vi "Query_Pelletron_Status.vi"(8 "error in (no error)":errorcluster, 10 "Read Selector":T1 items=["Facility Key", "Chain Bypass", "Rotating Shaft Bypass", "Facility Interlock", "Pressure Interlock", "Temperature Interlock", "Water Flow Interlock", "Blower Status", "High Voltage", "+ High Voltage PS Readout", "- High Voltage PS Readout", "High Voltage PS Setting", "Ion Gauge", "Ion Filament", "Control Reference Voltage", "Control Mode", "Power Supply", "Chain Current", "Column Current", "Lost Current", "High Voltage Power Supply", "Rotating Shaft", "Chain", "Beamline GV", "Radiation", "Spark Count", "Spark Limit", "Spark Interlock", "Spark Threshold", "HV Difference from Control"], 11 "AccelNET.lvlib:TCP.lvclass":refnum<class "TCP.lvclass">) -> (0 "error out":errorcluster, 2 "Data Out":dbl)   [LabVIEW 2012, in "AccelNET.lvlib" / "TCP.lvclass"]
uses:
  TCP.lvclass
  Read_Selector.ctl
  TCP.lvclass/TCP.ctl
  Useful_Controls.lvlib
panel:
  out "substring":string
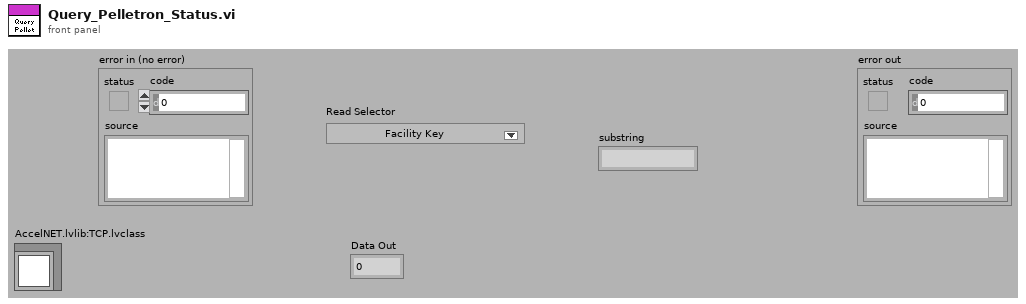
[diagram p1: front panel]
types:
  T1 = typedef "AccelNET.lvlib/Useful_Controls.lvlib/Read_Selector.ctl" = u16
  T2 = enum16{"Standard", "Buffered", "CRLF", "Immediate"}
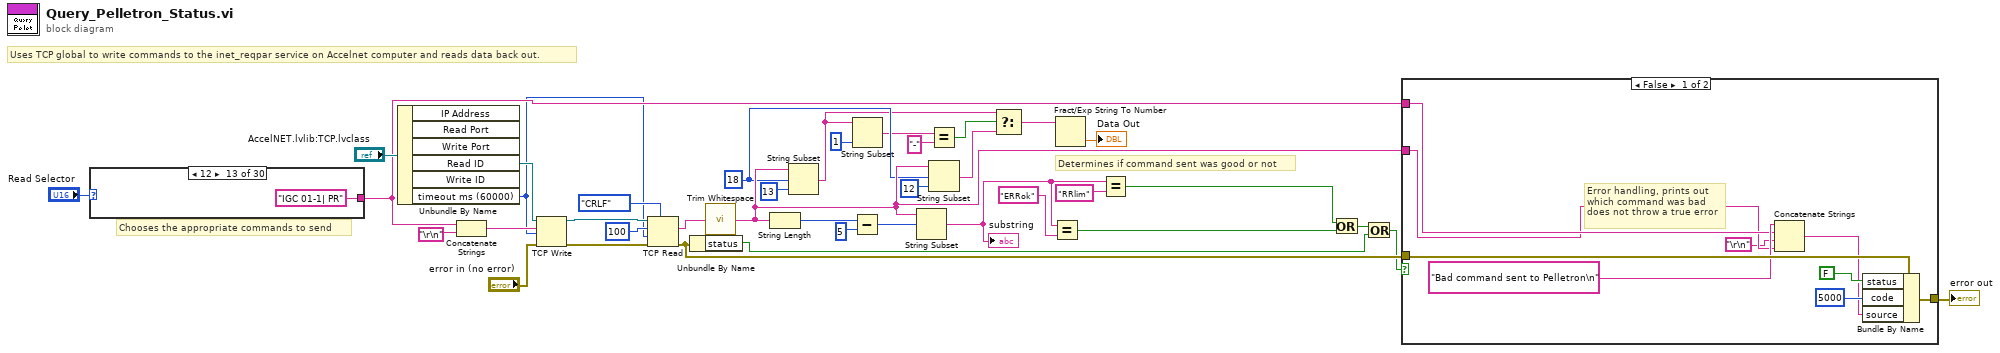
[diagram p0: block diagram]
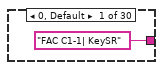
[diagram p3: hidden frame]
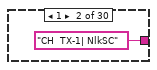
[diagram p4: hidden frame]
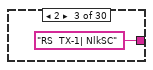
[diagram p5: hidden frame]
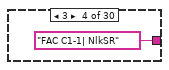
[diagram p6: hidden frame]
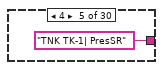
[diagram p7: hidden frame]
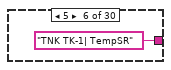
[diagram p8: hidden frame]
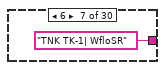
[diagram p9: hidden frame]
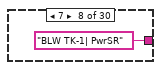
[diagram p10: hidden frame]
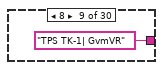
[diagram p11: hidden frame]
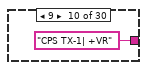
[diagram p12: hidden frame]
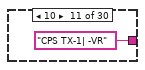
[diagram p13: hidden frame]
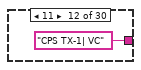
[diagram p14: hidden frame]
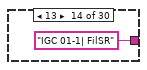
[diagram p15: hidden frame]
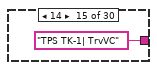
[diagram p16: hidden frame]
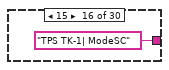
[diagram p17: hidden frame]
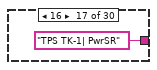
[diagram p18: hidden frame]
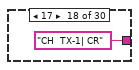
[diagram p19: hidden frame]
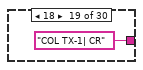
[diagram p20: hidden frame]
diagram:
  w9 = 18 ("offset (0)")
  # "Determines if command sent was good or not"
  # "Chooses the appropriate commands to send"
  # "Uses TCP global to write commands to the inet_reqpar service on Accelnet computer and reads data back out."
  n1 = case shown="12" "Read Selector" {
    tunnel: ["FAC C1-1| KeySR" "CH  TX-1| NlkSC" "RS  TX-1| NlkSC" "FAC C1-1| NlkSR" "TNK TK-1| PresSR" "TNK TK-1| TempSR" "TNK TK-1| WfloSR" "BLW TK-1| PwrSR" "TPS TK-1| GvmVR" "CPS TX-1| +VR" "CPS TX-1| -VR" "CPS TX-1| VC" "IGC 01-1| PR" "IGC 01-1| FilSR" "TPS TK-1| TrvVC" "TPS TK-1| ModeSC" "TPS TK-1| PwrSR" "CH  TX-1| CR" "COL TX-1| CR" "CH  TX-1| CRlost" "CPS TX-1| PwrSR" "RS  TX-1| PwrSC" "CH  TX-1| PwrSR" "BLV 01-1| PosSR" "RAD C1-1| VR" "SETUP| SparkCnt" "SETUP| SparkLim" "SETUP| EnableSC" "SETUP| SparkThr" "TPS TK-1| Gvm-Ref"] -> w24
    frame 0, Default {
    }
    frame 1 {
    }
    frame 2 {
    }
    frame 3 {
    }
    frame 4 {
    }
    frame 5 {
    }
    frame 6 {
    }
    frame 7 {
    }
    frame 8 {
    }
    frame 9 {
    }
    frame 10 {
    }
    frame 11 {
    }
    frame 12 {
    }
    frame 13 {
    }
    frame 14 {
    }
    frame 15 {
    }
    frame 16 {
    }
    frame 17 {
    }
    frame 18 {
    }
    frame 19 {
    }
    frame 20 {
    }
    frame 21 {
    }
    frame 22 {
    }
    frame 23 {
    }
    frame 24 {
    }
    frame 25 {
    }
    frame 26 {
    }
    frame 27 {
    }
    frame 28 {
    }
    frame 29 {
    }
  }
  n2 = Unbundle By Name("AccelNET.lvlib:TCP.lvclass") -> ("Read ID"=w26:refnum<k5>, "timeout ms (60000)"=w19:i32)  [unwired: 4 out]
  n3 = Concatenate Strings(w24, "\r\n") -> (w36:string)
  n4 = TCP Write(connection ID=w26, data in=w36, error in (no error)="error in (no error)", 9:w19) -> (connection ID out=w35:refnum<k5>, error out=w34:errorcluster)  [unwired: 1 out]
  n5 = TCP Read(connection ID=w35, bytes to read=100, error in (no error)=w34, 7:T2."CRLF" ("mode (standard)"), 9:w19) -> (data out=w18:string, error out=w14:errorcluster)  [unwired: 1 out]
  n6 = Unbundle By Name(w14) -> ("status"=w11:bool)
  n7 = call <vilib>:"Trim Whitespace.vi"("string"=w18) -> ("trimmed string"=w10:string)  [unwired: 1 in]
  n8 = String Length(string=w10) -> (length=w17:i32)
  n9 = String Subset(string=w10, offset (0)=w9, length (rest)=13 ("length (rest)")) -> (substring=w3:string)
  n10 = Subtract(x=w17, y=5 ("length (rest)")) -> (x-y=w15:i32)
  n11 = String Subset(string=w3, length (rest)=1 ("length (rest)")) -> (substring=w6:string)  [unwired: 1 in]
  n12 = String Subset(string=w10, offset (0)=w15) -> (substring=w23:string)  [unwired: 1 in]
  "substring" <- w23
  n13 = Equal?(x=w6, y="-") -> (x = y?=w4:bool)
  n14 = String Subset(string=w10, offset (0)=w9, length (rest)=12 ("length (rest)")) -> (substring=w2:string)
  n15 = Select(t=w3, s=w4, f=w2) -> (s? t:f=w1:string)
  n16 = Equal?(x=w23, y="ERRok") -> (x = y?=w20:bool)
  n17 = Fract/Exp String To Number(string=w1) -> (number=→"Data Out":dbl)  [unwired: 3 in, 1 out]
  n18 = Equal?(x=w23, y="RRlim") -> (x = y?=w21:bool)
  n19 = Or(x=w21, y=w20) -> (x .or. y?=w12:bool)
  n20 = Or(x=w12, y=w11) -> (x .or. y?=w13:bool)
  n21 = case shown="False" w13 {
    tunnel: w14 -> [w77 w78]
    tunnel: [w75 w78] -> w25
    tunnel: w24 -> [w72 _]
    tunnel: w10 -> [w70 _]
    frame False {
      # "Error handling, prints out\nwhich command was bad\ndoes not throw a true error"
      n22 = Concatenate Strings("Bad command sent to Pelletron\n" ("source"), w72, "\r\n", w70) -> (w71:string)
      n23 = Bundle By Name(cluster=w77, "status"=FALSE, "code"=5000, "source"=w71) -> (w75:errorcluster)
    }
    frame True {
    }
  }
  "error out" <- w25
